vi "setMain.vi"(8 "error in (no error)":errorcluster, 10 "Main":T1={"Primary"=15224622, "Primary Variant"=16744512, "Secondary"=9342606, "Secondary Varient"=2039583}, 11 "Theme.Colors in":refnum<class "Theme.Colors.lvclass">) -> (0 "error out":errorcluster, 3 "Theme.Colors out":refnum<class "Theme.Colors.lvclass">)   [LabVIEW 2017, in "Theme.lvlib" / "Theme.Colors.lvclass"]
uses:
  Theme.Colors.lvclass
  Theme.Colors.lvclass/Theme.Colors.ctl
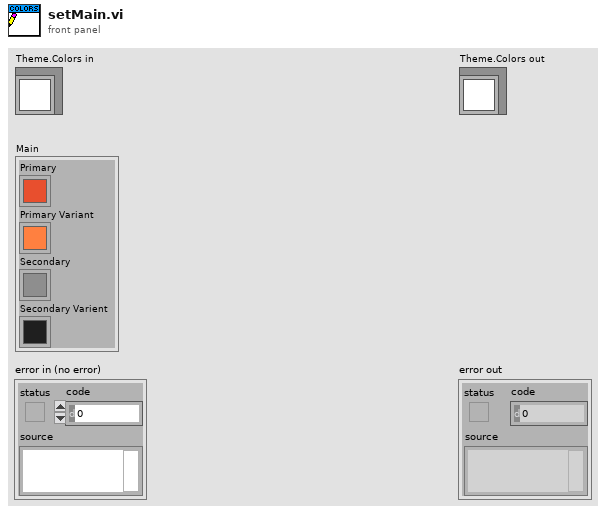
[diagram p1: front panel]
types:
  T1 = cluster{"Primary":u32, "Primary Variant":u32, "Secondary":u32, "Secondary Varient":u32}
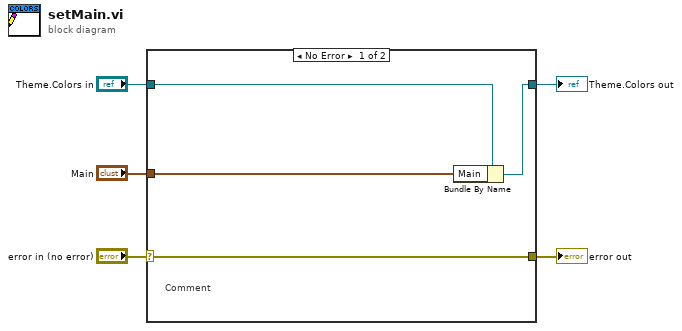
[diagram p0: block diagram]
diagram:
  n1 = case shown="No Error" "error in (no error)" {
    selector: "error in (no error)" -> [w9 w10]
    tunnel: [w9 w10] -> w4
    tunnel: [w7 w11] -> w2
    tunnel: "Theme.Colors in" -> [w8 w11]
    tunnel: "Main" -> [w6 _]
    frame No Error {
      # "Comment"
      n2 = Bundle By Name(cluster=w8, "Main"=w6) -> (w7:refnum<class "Theme.Colors.lvclass">)
    }
    frame Error {
    }
  }
  "error out" <- w4
  "Theme.Colors out" <- w2
